vi "Pull_Data_Client.vi"(2 "application reference":refnum<vi>, 3 "error in (no error)":errorcluster, 4 "Archive File?":bool, 5 "Running on Server?":bool, 6 "Path of File relative to EnFlo Data Root":path) -> (0 "error out":errorcluster)   [LabVIEW 2011]
uses:
  Anemometry/Anemometry Sub Vis/Globals/Constants_global.vi
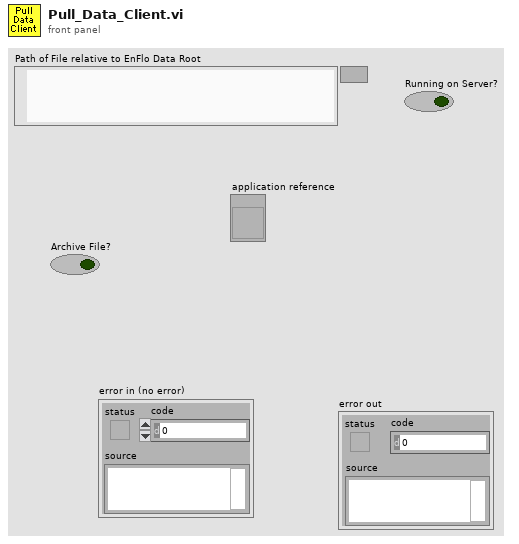
[diagram p1: front panel]
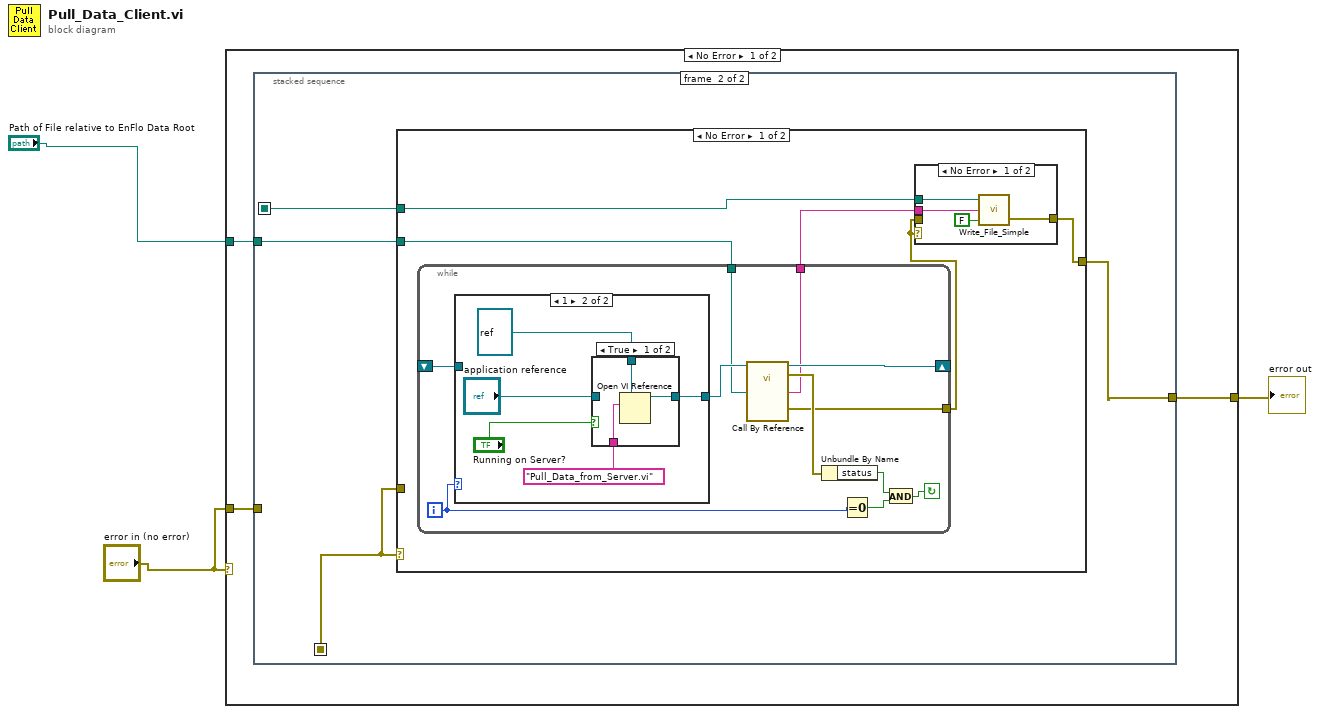
[diagram p0: block diagram]
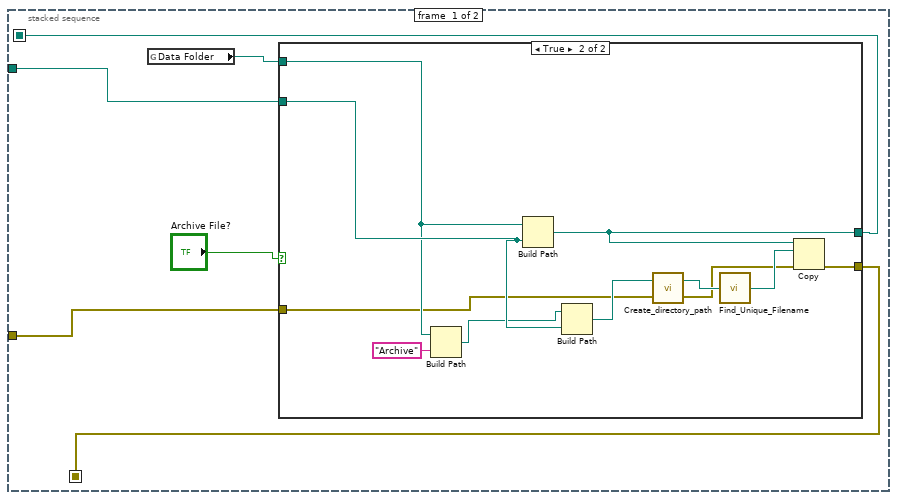
[diagram p2: hidden frame]
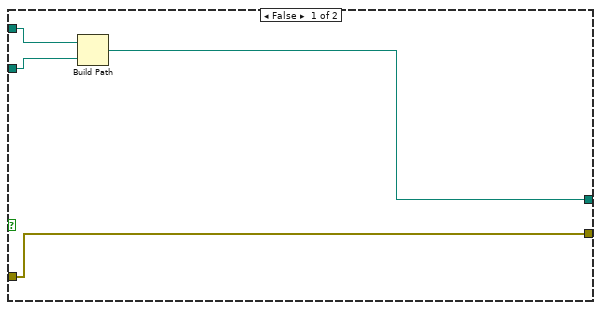
[diagram p3: hidden frame]
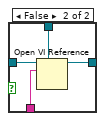
[diagram p6: hidden frame]
diagram:
  n1 = case shown="No Error" "error in (no error)" {
    tunnel: [w6 w67] -> w3
    tunnel: "error in (no error)" -> [w5 w67]
    tunnel: "Path of File relative to EnFlo Data Root" -> [w4 _]
    frame No Error {
      n2 = stacked-sequence {
        seq-local: [w9 _] -> [_ w28]
        seq-local: [w8 _] -> [_ w30]
        tunnel: [_ w31] -> w6
        tunnel: w5 -> [w10 _]
        tunnel: w4 -> [w7 w29]
        frame #0 {
          n3 = global read "Constants_global.vi" "Data Folder"() -> (w12:path)
          n4 = case shown="True" "Archive File?" {
            tunnel: w12 -> [w16 w21]
            tunnel: w7 -> [w15 w23]
            tunnel: [w13 w19] -> w9
            tunnel: w10 -> [w13 w18]
            tunnel: [w14 w17] -> w8
            frame False {
              n5 = Build Path(base path=w16, name or relative path=w15) -> (appended path=w14:path)
            }
            frame True {
              n6 = Build Path(base path=w21, name or relative path="Archive") -> (appended path=w20:path)
              n7 = Build Path(base path=w21, name or relative path=w23) -> (appended path=w17:path)
              n8 = Build Path(base path=w20, name or relative path=w23) -> (appended path=w26:path)
              n9 = call "Create_directory_path.vi"("error in (no error)"=w18, "Path name"=w26) -> ("error out"=w24:errorcluster, "Path name Out"=w25:path)
              n10 = call "Find_Unique_Filename.vi"("Path In"=w25) -> ("Unique Path Out"=w27:path)  [unwired: 2 in]
              n11 = Copy(8:w24, 10:w27, 11:w17) -> (0:w19:errorcluster)  [unwired: 2 in, 2 out]
            }
          }
        }
        frame #1 {
          n12 = case shown="No Error" w28 {
            tunnel: [w33 w66] -> w31
            tunnel: w28 -> [_ w66]
            tunnel: w30 -> [w34 _]
            tunnel: w29 -> [w35 _]
            frame No Error {
              n13 = while {
                shift-right: [w50] -> _
                shift-left: _ -> [w52]
                tunnel: w35 -> [w44]
                tunnel: [w43] -> w36
                tunnel: [w42] -> w32
                i -> [w48]
                stop <- w45 continue-if-true
                n14 = case shown="1" w48 {
                  tunnel: w52 -> [w53 _]
                  tunnel: [w53 w58] -> w51
                  frame 0, Default {
                  }
                  frame 1 {
                    n15 = case shown="True" "Running on Server?" {
                      tunnel: [w61 w65] -> w58
                      tunnel: "application reference" -> [_ w64]
                      tunnel: refnum<vi> refnum ("Push Data Server") -> [w60 w63]
                      tunnel: "Pull_Data_from_Server.vi" -> [w59 w62]
                      frame True {
                        n16 = Open VI Reference(type specifier VI Refnum (for type only)=w60, vi path=w59) -> (vi reference=w61:refnum<vi>)  [unwired: 2 in, 3 out]
                      }
                      frame False {
                        n17 = Open VI Reference(type specifier VI Refnum (for type only)=w63, application reference (local)=w64, vi path=w62) -> (vi reference=w65:refnum<vi>)  [unwired: 1 in, 3 out]
                      }
                    }
                  }
                }
                n18 = call-by-ref "?"(reference=w51, "Path of File relative to EnFlo Data Root"=w44) -> (reference out=w50:refnum<vi>, error out=w49:errorcluster, "error out"=w42:errorcluster, "File String"=w43:string)  [unwired: 2 in]
                n19 = Unbundle By Name(w49) -> ("status"=w46:bool)
                n20 = Equal To 0?(x=w48) -> (x = 0?=w47:bool)
                n21 = And(x=w46, y=w47) -> (x .and. y?=w45:bool)
              }
              n22 = case shown="No Error" w32 {
                tunnel: w36 -> [w39 _]
                tunnel: w34 -> [w38 _]
                tunnel: [w37 w41] -> w33
                tunnel: w32 -> [_ w41]
                frame No Error {
                  n23 = call "Write_File_Simple.vi"("append to file? (new file:F)"=FALSE, "character string"=w39, "file path"=w38) -> ("error out"=w37:errorcluster)  [unwired: 1 out]
                }
                frame Error {
                }
              }
            }
            frame Error {
            }
          }
        }
      }
    }
    frame Error {
    }
  }
  "error out" <- w3
